vi "Image Processing.vi"() -> ()   [LabVIEW 2012]
uses:
  <vilib>/picture/picture.llb/Draw 8-Bit Pixmap.vi
  <vilib>/imath/engines/lvmath2/RunTimeEngine/ErrorHandling/NIMS_Finalize Error.vi
  <vilib>/imath/engines/lvmath2/RunTimeEngine/Managers/WorkSpace/UID Generator.vi
  <vilib>/imath/engines/lvmath2/RunTimeEngine/Managers/SymbolTable/Clear UID.vi
  <vilib>/imath/engines/lvmath2/RunTimeEngine/NodeEndStatement/NIMS_NodeEndStatement_Output.vi
  <instcachedir>/0/NIMS_NodeEndStatement_Output_53EC0D466D134D7ABD903AC30B43404B.lvgen/NIMS_NodeEndStatement_Output_53EC0D466D134D7ABD903AC30B43404B_011.vi
  <vilib>/imath/engines/lvmath2/RunTimeEngine/BuiltInFunctions/ones/NIMS_M=ones(I32,I32).vi
  <vilib>/imath/engines/lvmath2/RunTimeEngine/RunTimeType/NIMS_RunTimeType_From StrictType (excl LVString).vi
  <instcachedir>/0/NIMS_RunTimeType_From StrictType (excl LVString)_27CFCE38286AFF43ABD3E48A72A09368.lvgen/NIMS_RunTimeType_From StrictType (excl LVString)_27CFCE38286AFF43ABD3E48A72A09368_000.vi
  <vilib>/imathl/engines/lvmath/Functions/Error Handling/Create Error.vi
  <vilib>/imath/engines/lvmath2/RunTimeEngine/LocalVariableDefStatement/MC_LocalVariableDefStatement_Display.vi
  <vilib>/imath/engines/lvmath2/RunTimeEngine/BuiltInFunctions/conv2d/NIMS_conv2d(GM,GM,Str).vi
  <instcachedir>/0/NIMS_conv2d(GM,GM,Str)_C7D81E1B98E043D08C3460674E88E962.lvgen/NIMS_conv2d(GM,GM,Str)_C7D81E1B98E043D08C3460674E88E962_000.vi
  <vilib>/imath/engines/lvmath2/RunTimeEngine/BuiltInFunctions/uint8/NIMS_uint8(real).vi
  <instcachedir>/0/NIMS_uint8(real)_CAA419FBB1354DA296C59E18C46DECF0.lvgen/NIMS_uint8(real)_CAA419FBB1354DA296C59E18C46DECF0_001.vi
  <vilib>/imath/engines/lvmath2/RunTimeEngine/ErrorHandling/NIMS_Error From Error Code.vi
  <instcachedir>/0/NIMS_NodeEndStatement_Output_53EC0D466D134D7ABD903AC30B43404B.lvgen/NIMS_NodeEndStatement_Output_53EC0D466D134D7ABD903AC30B43404B_009.vi
  <vilib>/imath/engines/lvmath2/RunTimeEngine/BuiltInFunctions/abs/NIMS_abs(signed).vi
  <instcachedir>/0/NIMS_abs(signed)_C4FCB8E6058B49B797C7C8D53CA5F6EC.lvgen/NIMS_abs(signed)_C4FCB8E6058B49B797C7C8D53CA5F6EC_005.vi
  <vilib>/imath/engines/lvmath2/RunTimeEngine/RunTimeType/NIMS_RunTimeType_Set Source Original Bool.vi
  <vilib>/imath/engines/lvmath2/RunTimeEngine/BitwiseOperatorToken/NIMS_Bitwise_Operator_Or.vi
  <instcachedir>/0/NIMS_Bitwise_Operator_Or_ADFCAB76A2DABC48BC952D729C6F60E3.lvgen/NIMS_Bitwise_Operator_Or_ADFCAB76A2DABC48BC952D729C6F60E3_000.vi
  <vilib>/imath/engines/lvmath2/RunTimeEngine/Managers/SymbolTable/NIMS_WorkSpace.lvlib
panel:
  in  "Image Number 3":dbl
  out "Edges in Image 3":picture
  in  "Threshold":i32(slide) scale=0.0..10.0
  in  "Blur":i32(slide) scale=0.0..50.0
  in  "Image Number 2":dbl
  out "Blurred Image 2":picture
  in  "Image Number":dbl
  out "Origional Image":picture
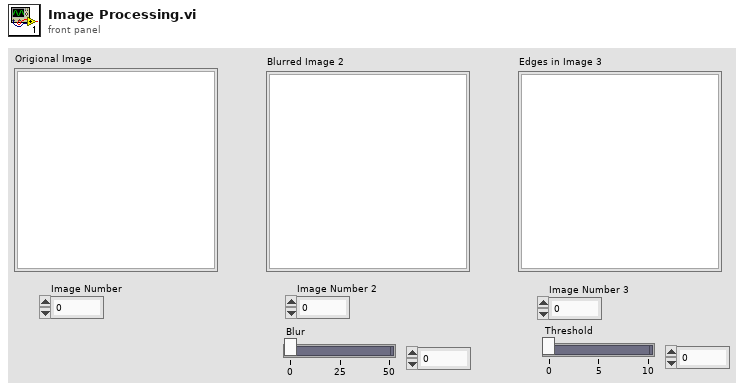
[diagram p1: front panel]
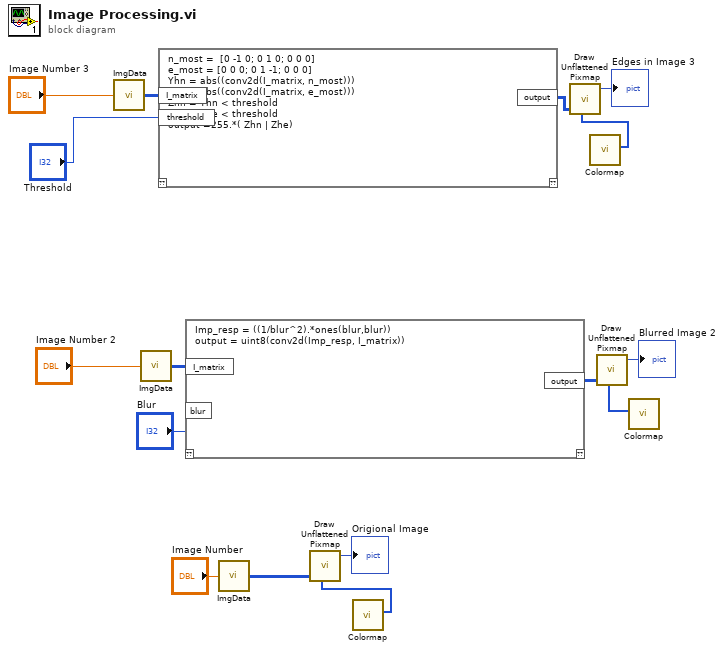
[diagram p0: block diagram]
diagram:
  n1 = call "ImgData.vi"("ImgNum"="Image Number 3") -> ("Data"=w3:u8[][])
  n2 = call "ImgData.vi"("ImgNum"="Image Number 2") -> ("Data"=w9:u8[][])
  n3 = mathscript code="n_most =  [0 -1 0; 0 1 0; 0 0 0]\ne_most = [0 0 0; 0 1 -1; 0 0 0]\nYhn = abs((conv2d(I_matrix, n_most))) \nYhe = abs((conv2d(I_matrix, e_most))) \nZhn = Yhn < threshold\nZhe = Yhe < threshold\noutput =255.*( Zhn | Zhe)"("I_matrix"=w3, "threshold"="Threshold") -> ("output"=w1:i32[][])  [unwired: 1 in, 1 out]
  n4 = mathscript code="Imp_resp = ((1/blur^2).*ones(blur,blur))\noutput = uint8(conv2d(Imp_resp, I_matrix))"("I_matrix"=w9, "blur"="Blur") -> ("output"=w8:u8[][])  [unwired: 1 in, 1 out]
  n5 = call "ImgData.vi"("ImgNum"="Image Number") -> ("Data"=w14:u8[][])
  n6 = call "Colormap.vi"() -> ("Array"=w16:u32[])  [unwired: 11 in]
  n7 = call-poly <vilib>:"Draw Unflattened Pixmap.vi"("data"=w14, "color table"=w16) -> ("new picture"=→"Origional Image":picture)  [unwired: 7 in]
  n8 = call "Colormap.vi"() -> ("Array"=w6:u32[])  [unwired: 11 in]
  n9 = call-poly <vilib>:"Draw Unflattened Pixmap.vi"("data"=w1, "color table"=w6) -> ("new picture"=→"Edges in Image 3":picture)  [unwired: 7 in]
  n10 = call "Colormap.vi"() -> ("Array"=w12:u32[])  [unwired: 11 in]
  n11 = call-poly <vilib>:"Draw Unflattened Pixmap.vi"("data"=w8, "color table"=w12) -> ("new picture"=→"Blurred Image 2":picture)  [unwired: 7 in]
